vi "Sub_Pin_Location.vi"() -> ()   [LabVIEW 2019]
panel:
  in  "Numeric":dbl
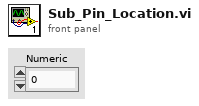
[diagram p1: front panel]
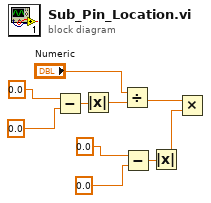
[diagram p0: block diagram]
diagram:
  n1 = Subtract(x=0.0, y=0.0) -> (x-y=w8:dbl)
  n2 = Absolute Value(x=w8) -> (abs(x)=w7:dbl)
  n3 = Divide(x="Numeric", y=w7) -> (x/y=w1:dbl)
  n4 = Subtract(x=0.0, y=0.0) -> (x-y=w4:dbl)
  n5 = Absolute Value(x=w4) -> (abs(x)=w2:dbl)
  n6 = Multiply(x=w1, y=w2) -> ()  [unwired: 1 out]
